vi "Save Buffer.vi"   [LabVIEW 2011, in "CAN FD.lvlib"]
uses:
  CAN FD.lvlib
types:
  T1 = enum16{"open", "replace", "create", "open or create", "replace or create", "replace or create with confirmation"}
  T2 = typedef "CAN FD.lvlib/CAN Data.ctl" = cluster{"SystemTime":timestamp, "HwTime":dbl, "Channel":u8, "ID":u32, "CANType":i16, "Direction":i16, "Remote":bool, "Ext":bool, "Len":u8, "Data":u8[], "Success":bool}
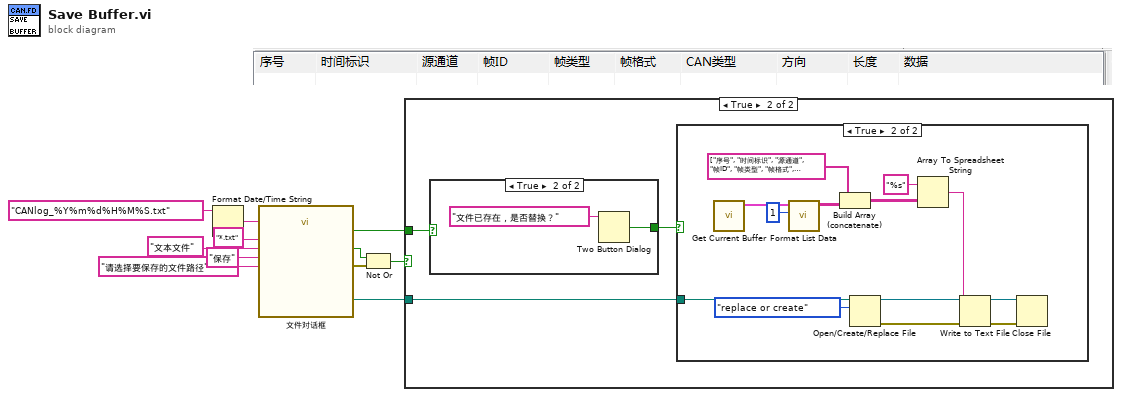
[diagram p0: block diagram]
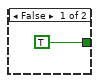
[diagram p4: hidden frame]
diagram:
  n1 = Format Date/Time String(time format string (%c)="CANlog_%Y%m%d%H%M%S.txt" ("时间格式字符串(%c)")) -> (date/time string=w10:string)  [unwired: 2 in]
  n2 = call "文件对话框"("prompt"="请选择要保存的文件路径", "button label"="保存", "default name"=w10, "pattern (all files)"="*.txt" ("pattern label"), "pattern label"="文本文件" ("pattern (all files)")) -> ("selected path"=w4:path, "exists"=w3:bool, "cancelled"=w6:bool, "error out"=w7:errorcluster)  [unwired: 7 in]
  n3 = Not Or(1:w7, 2:w6) -> (0:w5:bool)
  n4 = case shown="True" w5 {
    tunnel: w4 -> [_ w12]
    tunnel: w3 -> [_ w14]
    frame False {
    }
    frame True {
      n5 = case shown="True" w14 {
        tunnel: [TRUE ("T button?") w29] -> w13
        frame False {
        }
        frame True {
          n6 = Two Button Dialog(message="文件已存在，是否替换？" ("消息")) -> (T button?=w29:bool)  [unwired: 2 in]
        }
      }
      n7 = case shown="True" w13 {
        tunnel: w12 -> [_ w23]
        frame False {
        }
        frame True {
          n8 = call "Get Current Buffer.vi"() -> ("Data"=w27:T2[])  [unwired: 10 in, 1 out]
          n9 = call "Format List Data.vi"("#Offset"=1, "Data"=w27) -> ("List Data"=w25:string[][])  [unwired: 9 in]
          n10 = Build Array (concatenate)(string[] ["序号", "时间标识", "源通道", "帧ID", "帧类型", "帧格式", "CAN类型", "方向", "长度", "数据"], w25) -> (w19:string[][])
          n11 = Open/Create/Replace File(file path (use dialog)=w23, operation (0:open)=T1."replace or create" ("操作(0:open)")) -> (refnum out=w21:refnum<file>, error out=w20:errorcluster)  [unwired: 4 in, 1 out]
          n12 = Array To Spreadsheet String(array=w19, 3:"%s" ("格式字符串")) -> (spreadsheet string=w17:string)  [unwired: 1 in]
          n13 = Write to Text File(file (use dialog)=w21, text=w17, error in=w20) -> (refnum out=w15:refnum<file>, error out=w16:errorcluster)  [unwired: 1 in, 1 out]
          n14 = Close File(refnum=w15, error in=w16) -> ()  [unwired: 2 out]
        }
      }
    }
  }
